vi "Read Status.vi"(11 "channel":T1) -> (0 "Pending Write":i32[](array[numeric]), 1 "Pending Read":i32[](array[numeric]), 2 "Usage Ratio":dbl[](array[numeric]), 3 "Queued Count":i32[](array[numeric]), 4 "Closed?":bool, 5 "Updated":timestamp, 6 "Lossy":bool, 7 "Sequence":u32, 8 "Events":bool)   [LabVIEW 2022 SP3, in "Flex.lvlib"]
doc: "Does not return values from the channel but reads the status of the channel and reads the queue status for all the queues used with lossless readers. This endpoint does not return values from the channel, just the status."
uses:
  Flex.lvlib
  ))Channel.ctl
  Element.ctl
  ChannelOp.ctl
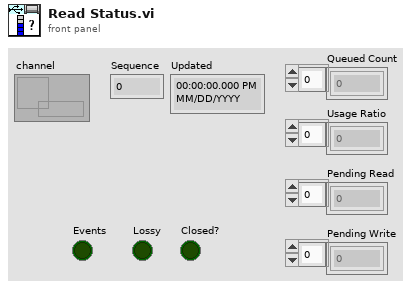
[diagram p1: front panel]
types:
  T1 = typedef "Flex.lvlib/))Channel.ctl" = refnum<queue>
  T2 = typedef "Flex.lvlib/ChannelOp.ctl" = enum16{"Get Refs", "Init", "Close", "Probe", "New Queue", "Remove Queue", "New Event"}
  T3 = typedef "Flex.lvlib/Channel Data.ctl" = cluster{"Event":refnum<user-event>, "Writer Ref":refnum<data-value>, "Lossy Queue":refnum<queue>}
  T4 = typedef "Flex.lvlib/Element Info.ctl" = cluster{"Value":T5, "Updated":timestamp, "Sequence":u32, "Paused":bool}
  T5 = typedef "Flex.lvlib/Element.ctl" = dbl
  T6 = typedef "Flex.lvlib/Writer Data.ctl" = cluster{"Lossless":refnum<queue>[], "Events":bool, "Lossy":bool}
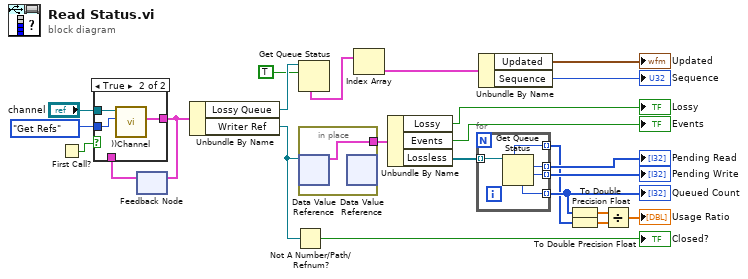
[diagram p0: block diagram]
diagram:
  n1 = First Call?() -> (First Call?: T/F=w23:bool)
  n2 = feedback #1() -> (w24:T3)  [unwired: 1 in]
  n3 = case shown="True" w23 {
    tunnel: w24 -> [w25 _]
    tunnel: [w25 w28] -> w20
    tunnel: "channel" -> [_ w27]
    tunnel: ChannelOp."Get Refs" ("channelOp") -> [_ w26]
    frame False {
    }
    frame True {
      n4 = call "))Channel.vi"("channelOp"=w26, "channel in"=w27) -> ("Channel Data"=w28:T3)  [unwired: 5 in, 4 out]
    }
  }
  n5 = feedback-in #1(w20) -> ()
  n6 = Unbundle By Name(w20) -> ("Lossy Queue"=w4:refnum<queue>, "Writer Ref"=w14:refnum<data-value>)
  n7 = Not A Number/Path/Refnum?(number/path/refnum=w14) -> (NaN/Path/Refnum?=→"Closed?":bool)
  n8 = Get Queue Status(queue=w4, return elements? (F)=TRUE) -> (elements=w2:T4[])  [unwired: 1 in, 7 out]
  n9 = in-place {
    in-place-border: [w29] -> w19
    n10 = in-place-dvr #2(w14) -> (w29:T6)  [unwired: 1 out]
    n11 = in-place-dvr #2() -> ()  [unwired: 1 in, 2 out]
  }
  n12 = Index Array(array=w2) -> (element=w1:T4)  [unwired: 1 in]
  n13 = Unbundle By Name(w19) -> ("Lossy"=→"Lossy":bool, "Events"=→"Events":bool, "Lossless"=w7:refnum<queue>[])
  n14 = for {
    tunnel: w7 -> [w34] mode=indexing
    tunnel: [w33] -> w12 mode=indexing
    tunnel: [w32] -> w18 mode=indexing
    tunnel: [w31] -> w17 mode=indexing
    tunnel: [w30] -> w11 mode=indexing
    n15 = Get Queue Status(queue=w34) -> (max queue size=w30:i32, # pending remove=w31:i32, # pending insert=w32:i32, # elements in queue=w33:i32)  [unwired: 2 in, 4 out]
  }
  "Queued Count" <- w12
  "Pending Write" <- w18
  "Pending Read" <- w17
  n16 = Unbundle By Name(w1) -> ("Updated"=→"Updated":timestamp, "Sequence"=→"Sequence":u32)
  n17 = To Double Precision Float(number=w12) -> (double precision float=w10:dbl[])
  n18 = To Double Precision Float(number=w11) -> (double precision float=w9:dbl[])
  n19 = Divide(x=w10, y=w9) -> (x/y=→"Usage Ratio":dbl[])
